vi "Send Send to Peer.vi"(5 "timeout ms (5000)":i32=5000, 7 "Priority":T2=enum."Normal" caption="Message Priority (Normal)", 8 "error in (no error)":errorcluster, 9 "Data Format (Text)":T1, 10 "Data":string, 11 "Message Enqueuer in":refnum<class "Message Enqueuer.lvclass">) -> (0 "error out":errorcluster, 3 "Message Enqueuer out":refnum<class "Message Enqueuer.lvclass">)   [LabVIEW 2021, in "WebSocket Actors.lvlib" / "Send to Peer Msg.lvclass"]
doc: "Sends the <b>WebSocket Actors.lvlib:Send to Peer Msg.lvclass</b> message.\n\nThis message will call <b>Send to Peer.vi</b> on the <b>WebSocket Actors.lvlib:WebSocket Connection.lvclass</b> actor.\n\n<b>Send to Peer.vi Description</b>\nThis method sends data to the connected peers in either text or binary format"
uses:
  Send to Peer Msg.lvclass
  <vilib>/ActorFramework/Message Enqueuer/Message Enqueuer.lvclass
  <vilib>/ActorFramework/Message Enqueuer/Message Priority.ctl
  LV-Websockets/Data Format.ctl
  C:/Program Files/National Instruments/LabVIEW 2021/vi.lib/ActorFramework/Message/Message.lvclass
  Send to Peer Msg.lvclass/Send to Peer Msg.ctl
  <vilib>/ActorFramework/Message Enqueuer/Message Enqueuer.lvclass/Message Enqueuer.ctl
  <vilib>/ActorFramework/Message Priority Queue/Priority Enqueue.vi
  LV-Websockets/LV WebSockets.lvlib
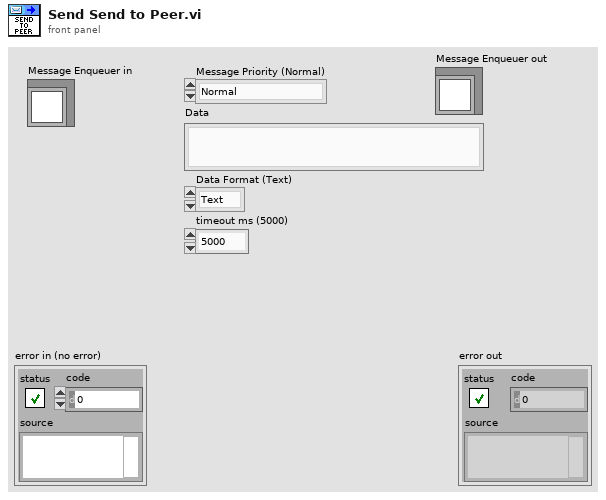
[diagram p1: front panel]
types:
  T1 = typedef "LV WebSockets.lvlib/Data Format.ctl" = enum16{"Text", "Binary"}
  T2 = typedef "Actor Framework.lvlib/Message Enqueuer.lvclass/Message Priority.ctl" = enum16{"Low", "Normal", "High"}
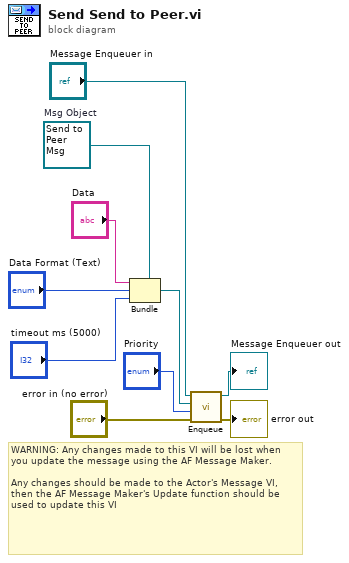
[diagram p0: block diagram]
diagram:
  w7 = refnum<class "Send to Peer Msg.lvclass"> refnum  # Msg Object
  # "WARNING: Any changes made to this VI will be lost when you update the message using the AF Message Maker.\n\nAny changes should be made to the Actor's Message VI, then the AF Message Maker's Update function should be used to update this VI"
  n1 = Bundle(cluster=w7, "Data", "Data Format (Text)", "timeout ms (5000)") -> (w2:refnum<class "Send to Peer Msg.lvclass">)
  n2 = call <vilib>:"Enqueue.vi"("error in (no error)"="error in (no error)", "Message Priority (Normal)"="Priority", "Message"=w2, "Message Enqueuer in"="Message Enqueuer in") -> ("error out"=→"error out":errorcluster, "Message Enqueuer out"=→"Message Enqueuer out":refnum<class "Message Enqueuer.lvclass">)  [unwired: 6 in]
